vi "Get Bind Port.vi"(8 "error in (no error)":errorcluster, 11 "Server Config in":refnum<class "Server Config.lvclass">) -> (0 "error out":errorcluster, 2 "Bind Port":u16, 3 "Server Config out":refnum<class "Server Config.lvclass">)   [LabVIEW 2020, in "Examples.lvlib" / "Server Config.lvclass"]
uses:
  Server Config.lvclass
  Server Config.lvclass/Server Config.ctl
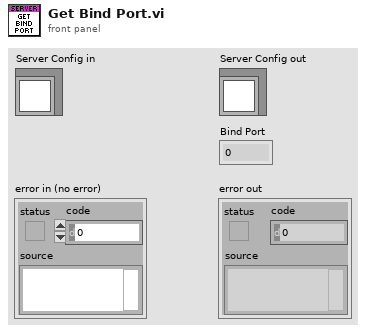
[diagram p1: front panel]
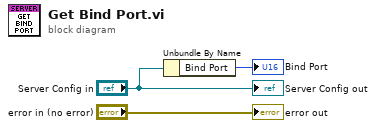
[diagram p0: block diagram]
diagram:
  n1 = Unbundle By Name("Server Config in") -> ("Bind Port"=→"Bind Port":u16)
  "error out" <- "error in (no error)"
  "Server Config out" <- "Server Config in"
